vi "USRP Dummy DMA Zero Copy (Host).vi"() -> ()   [LabVIEW 2016]
uses:
  <vilib>/userdefined/High Color/nirio_resource_hc.ctl
  <vilib>/FPGAPlugInAG/USRP 294xR; 295xR 200 MSps/niLvFpga_Open_USRP 294xR; 295xR 200 MSps.vi
  <vilib>/rvi/interface/common/dynamic/niFpgaDynamicAddResources.vi
  <vilib>/FPGAPlugInAG/Dynamic/niLvFpga_Download_Dynamic.vi
  <vilib>/FPGAPlugInAG/Dynamic/niLvFpga_Run_Dynamic.vi
  <vilib>/Utility/error.llb/Error Cluster From Error Code.vi
  <vilib>/rvi/errors/niLvFpgaAdjustHostInterfaceError.vi
  <vilib>/rvi/interface/common/niFpgaWaitOnOcc.vi
  <vilib>/FPGAPlugInAG/Dynamic/niLvFpga_Close_Dynamic.vi
  <vilib>/rvi/interface/nirviOpenFPGA/nirviOpenFPGA.xnode
  Bitfiles/USRP-RIO-Streami_DummyDMA_USRPDummy(FPGA)_kay5ptBR-r4.lvbitx
  <vilib>/rvi/interface/nirviMethod/nirviMethod.xnode
  <vilib>/rvi/interface/nirviReadWriteControl/nirviReadWriteControl.xnode
  <vilib>/rvi/interface/nirviCloseFPGA/nirviCloseFPGA.xnode
  <vilib>/rvi/errors/niLvFpgaMergeErrorWithErrorCode.vi
  <vilib>/rvi/interface/Simulation/niFpgaSimulationCallBeginRW.vi
  <instrlib>/niUsrpRio/Config/v1/Host/niUsrpRio Config v1 Host.lvlib
  NiFpgaLv.dll
  <vilib>/FPGAPlugInAG/Dynamic/niLvFpga_StopFifo_Dynamic.vi
  <vilib>/FPGAPlugInAG/Dynamic/niLvFpga_ConfigureFifo_Dynamic.vi
  <vilib>/FPGAPlugInAG/Dynamic/niLvFpga_StartFifo_Dynamic.vi
  <vilib>/FPGAPlugInAG/Dynamic/niLvFpga_AcquireReadRegionFifo_Dynamic.vi
panel:
  out "Random Generator":u64
  in  "Decimate (200 MHz)":u32=4
  in  "file path":path=path "C:/Users/jfernand/Desktop/USRP-RIO-Streaming/Streams/Dummy-DMA-TDMS-Test-File.tdms"
  out "Host Transfer Slider":u64(slide) scale=0.0..1073741824.0
  in  "Flush FIFO?":bool
  out "Control Loop":i32
  in  "Host FIFO Fetch":u64=131072
  in  "Reset Host Count?":bool
  in  "Stop Transfer?":bool
  in  "Reset FPGA Count?":bool
  out "FPGA Side FIFO":cluster{u32, u32}(slide)={66, 63} scale=0.0..2047.0
  out "Host TDMS Buffer":cluster{u32, u32}(slide) scale=0.0..67108863.0
  out "Data Loop":i32
  out "Fetch Loop":i32
  out "Host Count":u64
  in  "Number of Samples":u64=1073741824
  out "FPGA Count":u64
  in  "Start Transfer":bool
  in  "terminate":bool
  out "Elements Remaining":u32
  out "Data":u64[](array[numeric]) format="%016x"
  out "Timeout Counts":u64
  in  "Reset Timeouts?":bool
  out "Actual Depth":u32
  in  "Host Requested Depth":u32=67108864
  out "error out":errorcluster
  in  "resource name":T1="PXI2Slot18Port1Dev1"
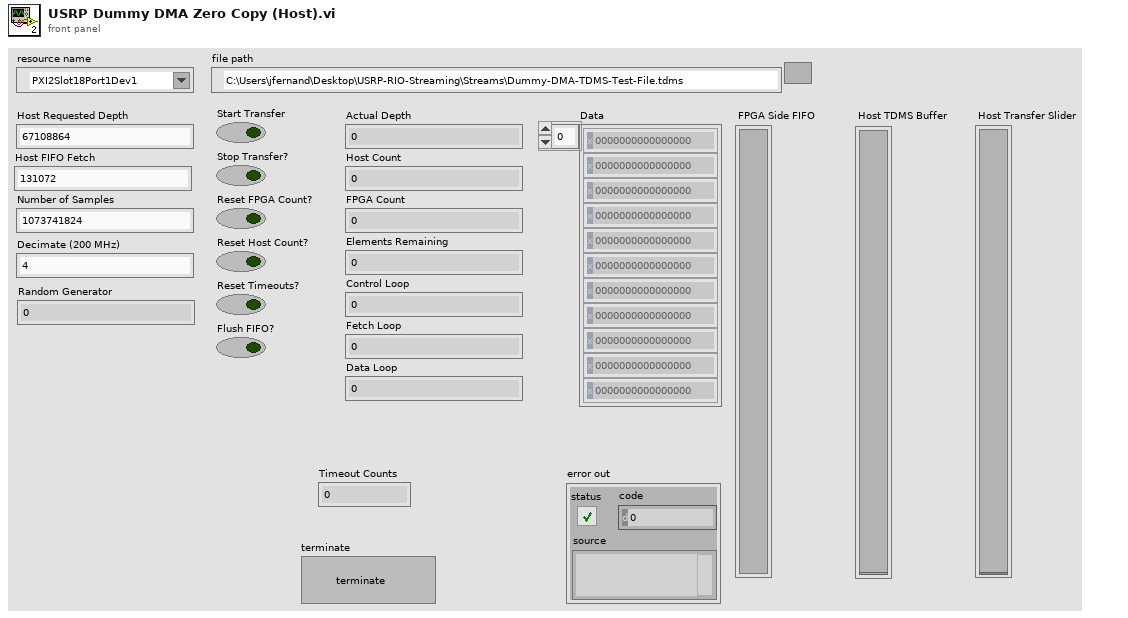
[diagram p1: front panel]
types:
  T1 = typedef "nirio_resource_hc.ctl" = tag
  T2 = enum16{"open", "open or create", "create or replace", "create", "open (read-only)"}
  T3 = typedef "niUsrpRio Config v1 Host.lvlib/niUsrpRio Session.ctl" = cluster{"FPGA Interface":refnum<k20>, "RIO Interface Number":u32, "Data Clock Rate":u32, "FPGA Data Clock Rate":u32, "Global Settings Register Bus":T4, "Radio 0 Settings Register Bus":T4, "Radio 1 Settings Register Bus":T4, "Radio Settings Bus Semaphore":T5, "DB Queues":T6[], "Characterization Data Valid?":bool, "EEPROM Header":T7, "Device Data Header":T8, "EEPROM Characterization Header":T9, "Characterization Data":T10[], "FPGA Current Version":u32, "FPGA Oldest Compatible Version":u32, "Fixed Logic Current Version":u32, "Fixed Logic Oldest Compatible Version":u32, "FPGA Radio Settings Bus Current Version":u32, "FPGA Radio Settings Bus Oldest Compatible Version":u32, "FPGA Board Config Current Version":u32, "FPGA Board Config Oldest Compatible Version":u32, "Daughterboard Clock Rate":u32, "daughterboard configuration session handles":u64[]}
  T4 = typedef "niInstr Register Bus v0 Host.lvlib/Register Bus Session.ctl" = refnum<queue>
  T5 = typedef "Semaphore RefNum" = refnum<k1>
  T6 = typedef "niUsrpRio Config v1 Host.lvlib/DB Queue Reference.ctl" = refnum<queue>
  T7 = typedef "niUsrpRio Config v1 Host.lvlib/EEPROM Header.ctl" = cluster{"Checksum":u32, "Product Code":u16, "Hardware Current Version":u16, "Hardware Oldest Compatible Version":u16, "EEPROM Map Current Version":u16, "EEPROM Map Oldest Compatible Version":u16, "User Password":string, "Pointer to Factory Header":u32, "Pointer to User Header":u32, "Recommended Interval":u16, "Number of Reserved Bytes":i32, "Number of Daughterboards":u8, "Daughterboard IDs":u16[], "Daughterboard Serial Numbers":string[]}
  T8 = typedef "niUsrpRio Config v1 Host.lvlib/EEPROM Device Data Header.ctl" = cluster{"Checksum":u32, "Number of Channels":u8, "Number of Gain Settings":u16[], "Pointer to Characterization Data":u32[], "Number of Reserved Bytes":i32, "Number of Frequencies":u16[]}
  T9 = typedef "niUsrpRio Config v1 Host.lvlib/EEPROM Characterization Header.ctl" = cluster{"Checksum":u32, "Date":timestamp, "Temperature":sgl, "Misc. Info":string, "Pointer to Device Data Header":u32, "Number of Reserved Bytes":i32}
  T10 = typedef "niUsrpRio Config v1 Host.lvlib/Characterization Data.ctl" = cluster{"Gains[dB]":dbl[], "Frequencies [Hz]":dbl[], "IQ Imbalance Table":T11[], "Measured Gains[dB]":dbl[][]}
  T11 = typedef "niUsrpRio Config v1 Host.lvlib/IQ Imbalance.ctl" = cluster{"Gain Imbalance [linear]":dbl, "Phase Imbalance [radians]":dbl, "Offset":cdb}
  T12 = cluster{"Running Max":u32, "Elements Remaining":u32}
  T13 = cluster{"Maximum Amount Used":u32, "Current Amount Used":u32}
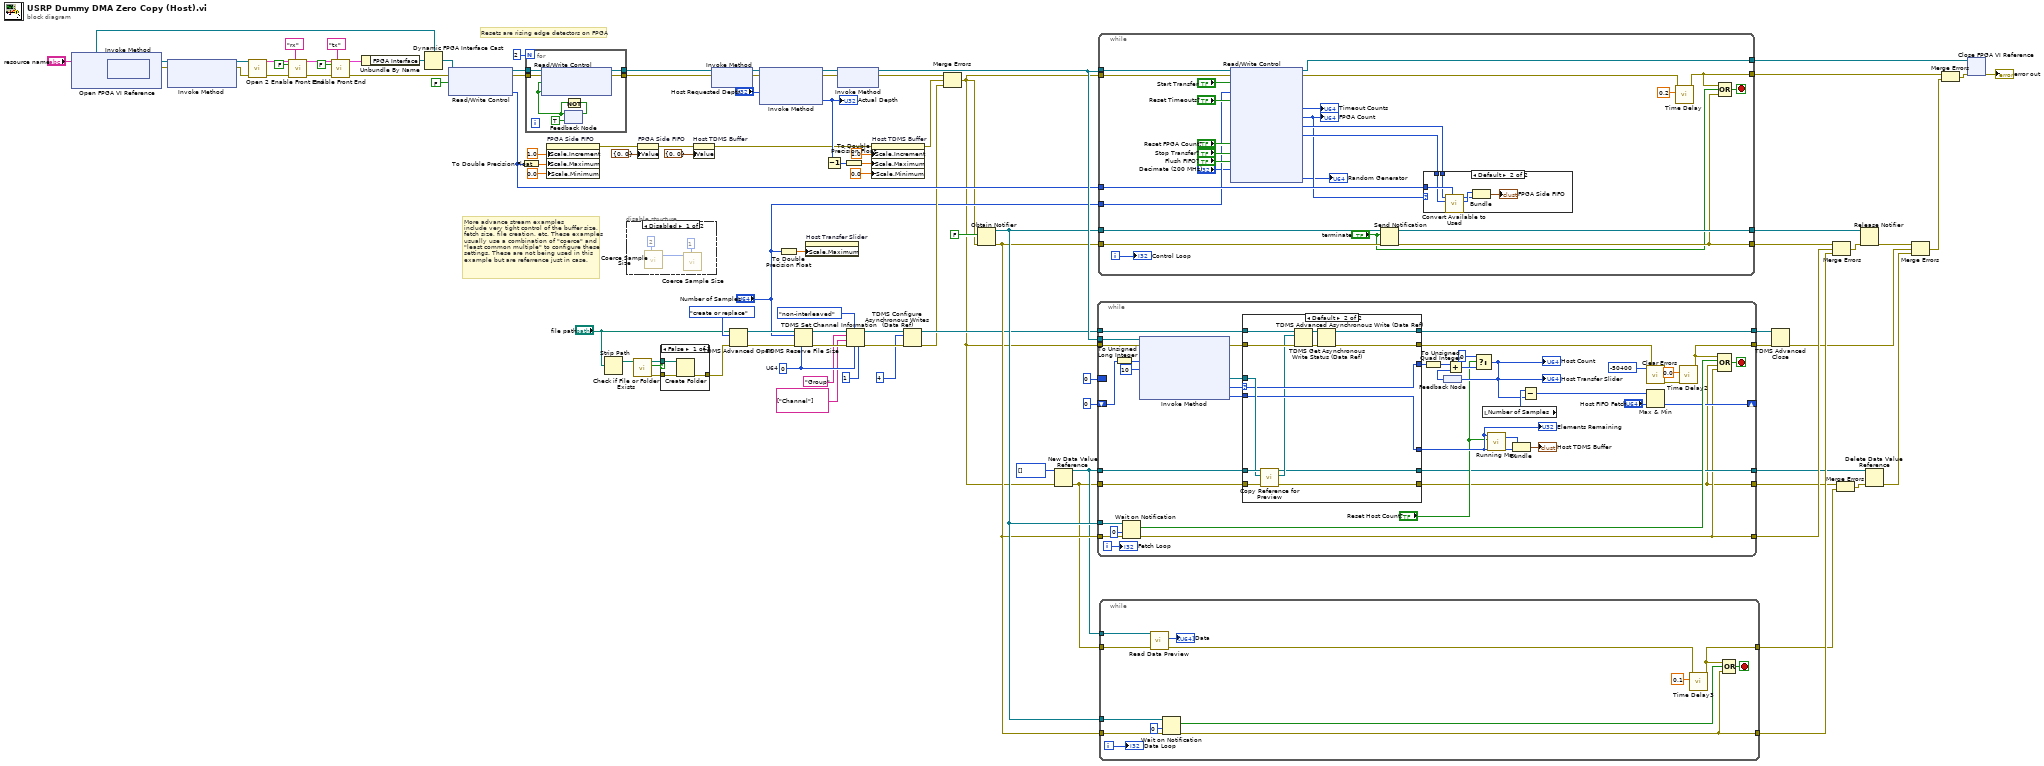
[diagram p0: block diagram]
diagram:
  w29 = u64 0  # U64
  # "More advance stream examples\ninclude very tight control of the buffer size,\nfetch size, file creation, etc. These examples\nusually use a combination of \"coerce\" and\n\"least common multiple\" to configure these\nsettings. These are not being used in this\nexample but are referrence just in case."
  # "Resets are rising edge detectors on FPGA"
  n1 = xnode "Open FPGA VI Reference"("resource name"="resource name") -> ("FPGA VI Reference Out"=w41:refnum<k20>, "error out"=w40:errorcluster)  [unwired: 1 in]
  n2 = xnode "Invoke Method"("FPGA VI Reference In"=w41, "error in"=w40) -> ("FPGA VI Reference Out"=w39:refnum<k20>, "error out"=w38:errorcluster)
  n3 = xnode "Invoke Method"("FPGA VI Reference In"=w39, "error in"=w38) -> ("FPGA VI Reference Out"=w37:refnum<k20>, "error out"=w36:errorcluster)  [unwired: 1 in]
  n4 = call <instrlib>:"Open 2.vi"("fpga ref"=w37, "error in"=w36) -> ("niUsrpRio Session (out)"=w87:T3, "error out"=w92:errorcluster)  [unwired: 12 in]
  n5 = call <instrlib>:"Enable Front End.vi"("niUsrpRio Session"=w87, "scope"="rx", "enable"=FALSE, "error in"=w92) -> ("niUsrpRio Session (out)"=w88:T3, "error out"=w91:errorcluster)  [unwired: 10 in]
  n6 = call <instrlib>:"Enable Front End.vi"("niUsrpRio Session"=w88, "scope"="tx", "enable"=FALSE, "error in"=w91) -> ("niUsrpRio Session (out)"=w84:T3, "error out"=w83:errorcluster)  [unwired: 10 in]
  n7 = Unbundle By Name(w84) -> ("FPGA Interface"=w82:refnum<k20>)
  n8 = Dynamic FPGA Interface Cast(Session In=w41, Type=w82) -> (Session Out=w81:refnum<k20>)
  n9 = xnode "Read/Write Control"("FPGA VI Reference In"=w81, "error in"=w83, "Start Transfer?"=FALSE ("send data?")) -> ("FPGA VI Reference Out"=w67:refnum<k20>, "error out"=w66:errorcluster, "FPGA FIFO Depth"=w53:u32)
  n10 = To Double Precision Float(number=w53) -> (double precision float=w55:dbl)
  n11 = for {
    N: 2 -> [_]
    tunnel: w67 -> [w105]
    tunnel: w66 -> [w104]
    tunnel: [w103] -> w65
    tunnel: [w102] -> w64
    n12 = feedback #1(TRUE) -> (w100:bool)
    n13 = xnode "Read/Write Control"("FPGA VI Reference In"=w105, "error in"=w104, "Reset Timeouts?"=w100, "Reset FPGA Count?"=w100) -> ("FPGA VI Reference Out"=w103:refnum<k20>, "error out"=w102:errorcluster)
    n14 = Not(x=w100) -> (.not. x?=w99:bool)
    n15 = feedback-in #1(w99) -> ()
  }
  n16 = property on="FPGA Side FIFO" class="Slide (strict)"("Scale.Increment"=1.0 ("Scale.Range:Increment"), "Scale.Maximum"=w55, "Scale.Minimum"=0.0 ("Scale.Range:Minimum")) -> (error out=w48:errorcluster)  [unwired: 2 in, 1 out]
  n17 = Strip Path(path="file path") -> (stripped path=w4:path)  [unwired: 1 out]
  n18 = disable-structure shown="Disabled" {
    frame Disabled {
      n19 = call "Coerce Sample Size.vi"("Bytes Per Sample (B)"=u64 2) -> ("Coerced Size (samples)"=w108:u64)  [unwired: 6 in]
      n20 = call "Coerce Sample Size.vi"("Bytes Per Sample (B)"=u64 1, "Size (samples)"=w108) -> ()  [unwired: 5 in, 1 out]
    }
    frame Enabled {
    }
  }
  n21 = call <vilib>:"Check if File or Folder Exists.vi"("path"=w4) -> ("error out"=w3:errorcluster, "file or folder exists?"=w1:bool, "dup path"=w2:path)  [unwired: 8 in]
  n22 = property on="FPGA Side FIFO" class="Slide (strict)"(error in=w48, "Value"=cluster{u32, u32} {0, 0} ("FPGA Side FIFO")) -> (error out=w51:errorcluster)  [unwired: 1 in, 1 out]
  n23 = case shown="False" w1 {
    tunnel: [w111 w112] -> w5
    tunnel: w3 -> [w110 w112]
    tunnel: w2 -> [w109 _]
    frame False {
      n24 = Create Folder(path (use dialog)=w109, error in=w110) -> (error out=w111:errorcluster)  [unwired: 1 in, 2 out]
    }
    frame True {
    }
  }
  n25 = property on="Host TDMS Buffer" class="Slide (strict)"(error in=w51, "Value"=cluster{u32, u32} {0, 0} ("FPGA Side FIFO")) -> (error out=w47:errorcluster)  [unwired: 1 in, 1 out]
  n26 = xnode "Invoke Method"("FPGA VI Reference In"=w65, "error in"=w64) -> ("FPGA VI Reference Out"=w98:refnum<k20>, "error out"=w97:errorcluster)
  n27 = TDMS Advanced Open(8:w5, 10:T2."create or replace" ("operation (0:open)"), 11:"file path") -> (0:w32:errorcluster, 3:w33:refnum<k34>)  [unwired: 2 in, 1 out]
  n28 = xnode "Invoke Method"("FPGA VI Reference In"=w98, "error in"=w97, "Requested Depth"="Host Requested Depth") -> ("FPGA VI Reference Out"=w94:refnum<k20>, "error out"=w95:errorcluster, "Actual Depth"=w52:u32)
  "Actual Depth" <- w52
  n29 = To Double Precision Float(number="Number of Samples") -> (double precision float=w16:dbl)
  n30 = TDMS Reserve File Size(6:w29, 8:w32, 10:"Number of Samples", 11:w33) -> (0:w30:errorcluster, 3:w31:refnum<k34>)  [unwired: 1 in]
  n31 = property on="Host Transfer Slider" class="Slide (strict)"("Scale.Maximum"=w16) -> ()  [unwired: 2 in, 2 out]
  n32 = Decrement(x=w52) -> (x-1=w58:u32)
  n33 = xnode "Invoke Method"("FPGA VI Reference In"=w94, "error in"=w95) -> ("FPGA VI Reference Out"=w79:refnum<k20>, "error out"=w54:errorcluster)
  n34 = To Double Precision Float(number=w58) -> (double precision float=w42:dbl)
  n35 = TDMS Set Channel Information(4:u32 1 ("samples per channel"), 6:w29, 7:enum16{"non-interleaved", "interleaved"}."non-interleaved" ("data layout (0:non-interleaved)"), 8:w30, 9:string[] ["Channel"] ("channel name(s)"), 10:"Group" ("group name (Untitled)"), 11:w31) -> (0:w25:errorcluster, 3:w26:refnum<k34>)
  n36 = property on="Host TDMS Buffer" class="Slide (strict)"(error in=w47, "Scale.Increment"=1.0 ("Data Entry Limits:Increment"), "Scale.Maximum"=w42, "Scale.Minimum"=0.0 ("Data Entry Limits:Minimum")) -> (error out=w46:errorcluster)  [unwired: 1 in, 1 out]
  n37 = TDMS Configure Asynchronous Writes (Data Ref)(8:w25, 10:u32 4 ("max asynchronous writes (4)"), 11:w26) -> (0:w20:errorcluster, 3:w21:refnum<k34>)  [unwired: 1 in]
  n38 = Merge Errors(w54, w46, w20) -> (w12:errorcluster)
  n39 = Obtain Notifier(notification data type=FALSE, error in (no error)=w12) -> (notifier out=w71:refnum<notifier>, error out=w70:errorcluster)  [unwired: 2 in, 1 out]
  n40 = New Data Value Reference(data value=u64[] [] ("Data"), error in=w12) -> (data value reference=w13:refnum<data-value>, error out=w10:errorcluster)
  n41 = while {
    tunnel: [w148] -> w19
    tunnel: w79 -> [w151]
    tunnel: w12 -> [w150]
    border: u64 0 -> [_]
    tunnel: w71 -> [w144]
    tunnel: w70 -> [w143]
    tunnel: [w114] -> w73
    tunnel: w10 -> [w140]
    tunnel: [w113] -> w9
    shift-right: [w133] -> _
    shift-left: u64 0 -> [w134]
    tunnel: w21 -> [w126]
    tunnel: [w125] -> w18
    tunnel: w13 -> [w122]
    tunnel: [w115] -> w11
    i -> [w141]
    stop <- w146 stop-if-true
    n42 = To Unsigned Long Integer(number=w134) -> (unsigned 32bit integer=w132:u32)
    n43 = Wait on Notification(notifier=w144, timeout in ms (-1)=0, error in (no error)=w143) -> (notification=w142:bool, error out=w114:errorcluster)  [unwired: 1 in, 2 out]
    n44 = xnode "Invoke Method"("FPGA VI Reference In"=w151, "error in"=w150, "Number of Elements"=w132, "Timeout (ms)"=10) -> ("error out"=w128:errorcluster, "Read Region Reference"=w123:refnum<data-value>, "Elements In Region"=w124:u32, "Elements Remaining"=w121:u32)  [unwired: 1 out]
    n45 = case shown="Default" w124 {
      selector: w124 -> [w155 w162]
      tunnel: w140 -> [w157 w173]
      tunnel: [w157 w172] -> w113
      tunnel: w128 -> [w158 w171]
      tunnel: [w158 w170] -> w127
      tunnel: w121 -> [w156 w163]
      tunnel: w126 -> [w159 w169]
      tunnel: [w159 w168] -> w125
      tunnel: w123 -> [_ w164]
      tunnel: w122 -> [w154 w165]
      tunnel: [w156 w163] -> w117
      tunnel: [w155 w162] -> w120
      tunnel: [w154 w160] -> w115
      frame 0 {
      }
      frame Default {
        n46 = call "Copy Reference for Preview.vi"("error in (no error)"=w173, "FPGA FIFO Reference in"=w164, "Data Preview Reference in"=w165) -> ("error out"=w172:errorcluster, "FPGA FIFO Reference out"=w161:refnum<data-value>, "Data Preview Reference out"=w160:refnum<data-value>)  [unwired: 6 in]
        n47 = TDMS Advanced Asynchronous Write (Data Ref)(8:w171, 10:w161, 11:w169) -> (0:w166:errorcluster, 3:w167:refnum<k34>)  [unwired: 1 in]
        n48 = TDMS Get Asynchronous Write Status (Data Ref)(8:w166, 11:w167) -> (0:w170:errorcluster, 3:w168:refnum<k34>)  [unwired: 1 out]
      }
    }
    "Elements Remaining" <- w117
    n49 = To Unsigned Quad Integer(1:w120) -> (0:w153:u64)
    n50 = feedback #2() -> (w152:u64)
    n51 = Add(x=w153, y=w152) -> (x+y=w139:u64)
    n52 = Select(t=u64 0, s="Reset Host Count?", f=w139) -> (s? t:f=w136:u64)
    "Host Count" <- w136
    "Host Transfer Slider" <- w136
    n53 = feedback-in #2(w136) -> ()
    n54 = local read "Number of Samples"() -> (w137:u64)
    n55 = call "Running Max.vi"("Reset"="Reset Host Count?", "Next Value"=w117) -> ("Running Max"=w119:u32)  [unwired: 5 in]
    n56 = Bundle("Running Max"=w119, "Elements Remaining"=w117) -> (→"Host TDMS Buffer":T12)  [unwired: 1 in]
    n57 = Subtract(x=w137, y=w136) -> (x-y=w135:u64)
    n58 = call <vilib>:"Clear Errors.vi"("error in (no error)"=w127, "specific error code to clear (0: all)"=-50400) -> ("error out"=w131:errorcluster)  [unwired: 4 in, 1 out]
    n59 = Max & Min(x=w135, y="Host FIFO Fetch") -> (min(x,y)=w133:u64)  [unwired: 1 out]
    n60 = call "Time Delay2"("error in (no error)"=w131, "Delay Time (s)"=0.0) -> ("error out"=w148:errorcluster)  [unwired: 9 in]
    n61 = Compound Arithmetic op=OR(w148, w142, w113, w114) -> (w146:bool)
    "Fetch Loop" <- w141
  }
  n62 = while {
    tunnel: w79 -> [w199]
    tunnel: w12 -> [w198]
    tunnel: w71 -> [w195]
    tunnel: w70 -> [w194]
    tunnel: [w193] -> w76
    tunnel: [w192] -> w75
    tunnel: [w188] -> w63
    tunnel: [w187] -> w62
    tunnel: w53 -> [w186]
    tunnel: "Number of Samples" -> [w177]
    i -> [w179]
    stop <- w191 stop-if-true
    n63 = xnode "Read/Write Control"("FPGA VI Reference In"=w199, "error in"=w198, "Start Transfer?"="Start Transfer", "Number of Samples"=w177, "Reset Timeouts?"="Reset Timeouts?", "Reset Timeouts?"="Reset FPGA Count?", "Stop Transfer?"="Stop Transfer?", "Flush FIFO?"="Flush FIFO?", "Decimate (200MHz)"="Decimate (200 MHz)") -> ("FPGA VI Reference Out"=w187:refnum<k20>, "error out"=w197:errorcluster, "Timeout Count"=→"Timeout Counts":u64, "FPGA Count"=w180:u64, "Space Available"=w185:u32, "Min Space Available"=w183:u32, "Random Number"=→"Random Generator":u64)
    "FPGA Count" <- w180
    n64 = Send Notification(notification="terminate", notifier=w195, error in (no error)=w194) -> (notifier out=w193:refnum<notifier>, error out=w192:errorcluster)
    n65 = case shown="Default" w180 {
      tunnel: w186 -> [_ w205]
      tunnel: w185 -> [_ w204]
      tunnel: w183 -> [_ w203]
      frame 0 {
      }
      frame Default {
        n66 = call "Convert Available to Used.vi"("Size"=w205, "Minimum Amount Available"=w203, "Current Amount Available"=w204) -> ("Maximum Amount Used"=w202:u32, "Current Amount Used"=w201:u32)  [unwired: 5 in]
        n67 = Bundle("Maximum Amount Used"=w202, "Current Amount Used"=w201) -> (→"FPGA Side FIFO":T13)  [unwired: 1 in]
      }
    }
    n68 = call "Time Delay"("error in (no error)"=w197, "Delay Time (s)"=0.2) -> ("error out"=w188:errorcluster)  [unwired: 9 in]
    n69 = Compound Arithmetic op=OR(w188, "terminate", w192) -> (w191:bool)
    "Control Loop" <- w179
  }
  n70 = while {
    tunnel: w71 -> [w216]
    tunnel: w70 -> [w215]
    tunnel: [w210] -> w69
    tunnel: w13 -> [w209]
    tunnel: [w212] -> w68
    tunnel: w10 -> [w207]
    i -> [w218]
    stop <- w213 stop-if-true
    n71 = call "Read Data Preview.vi"("error in (no error)"=w207, "Data Value Reference in"=w209) -> ("error out"=w206:errorcluster, "Data"=→"Data":u64[])  [unwired: 7 in, 1 out]
    n72 = Wait on Notification(notifier=w216, timeout in ms (-1)=0, error in (no error)=w215) -> (notification=w214:bool, error out=w210:errorcluster)  [unwired: 1 in, 2 out]
    n73 = call "Time Delay3"("error in (no error)"=w206, "Delay Time (s)"=0.1) -> ("error out"=w212:errorcluster)  [unwired: 9 in]
    n74 = Compound Arithmetic op=OR(w212, w214, w210) -> (w213:bool)
    "Data Loop" <- w218
  }
  n75 = TDMS Advanced Close(8:w19, 11:w18) -> (0:w17:errorcluster)  [unwired: 2 in, 1 out]
  n76 = Merge Errors(w75, w73, w69) -> (w74:errorcluster)
  n77 = Merge Errors(w9, w68) -> (w8:errorcluster)
  n78 = Release Notifier(notifier=w76, error in (no error)=w74) -> (error out=w72:errorcluster)  [unwired: 1 in, 2 out]
  n79 = Delete Data Value Reference(data value reference=w11, error in=w8) -> (error out=w7:errorcluster)  [unwired: 1 out]
  n80 = Merge Errors(w72, w17, w7) -> (w43:errorcluster)
  n81 = Merge Errors(w63, w43) -> (w44:errorcluster)
  n82 = xnode "Close FPGA VI Reference"("FPGA VI Reference In"=w62, "error in"=w44) -> ("error out"=→"error out":errorcluster)
